vi "UltrasonicRead.vi"(0 "DIO Reference":T1, 1 "TimeoutMS":dbl, 3 "error in (no error)":errorcluster) -> (7 "DistanceM":dbl, 8 "Timeout":bool, 10 "error out":errorcluster)   [LabVIEW 2017]
uses:
  <vilib>/myRIO/Instrument Drivers/Onboard IO/DIO/typedefs/DIO Reference.ctl
  <vilib>/myRIO/Common/Instrument Driver Framework/Utilities/typedefs/myRIO Generic Hardware Reference.ctl
  <vilib>/myRIO/Common/Instrument Driver Framework/Utilities/typedefs/Hardware Version Enum.ctl
  <vilib>/myRIO/Common/Instrument Driver Framework/Utilities/typedefs/myRIO v1.0 Reference.ctl
  <vilib>/myRIO/Common/Instrument Driver Framework/Utilities/typedefs/Generic FPGA Reference.ctl
  <vilib>/myRIO/Common/Instrument Driver Framework/myRIO v1.0/DIO/typedefs/DIO Channels List.ctl
  <vilib>/myRIO/Common/Instrument Driver Framework/myRIO v1.0/DIO/typedefs/DIO Channels Enum.ctl
  <vilib>/Utility/error.llb/Error Cluster From Error Code.vi
  <vilib>/myRIO/Common/Instrument Driver Framework/myRIO v1.0/DIO/vis/myRIO v1.0 Write DIO.vi
  <vilib>/myRIO/Common/Instrument Driver Framework/myRIO v1.0/DIO/vis/myRIO v1.0 Read DIO.vi
  <vilib>/myRIO/Instrument Drivers/Onboard IO/DIO/DIO.lvlib
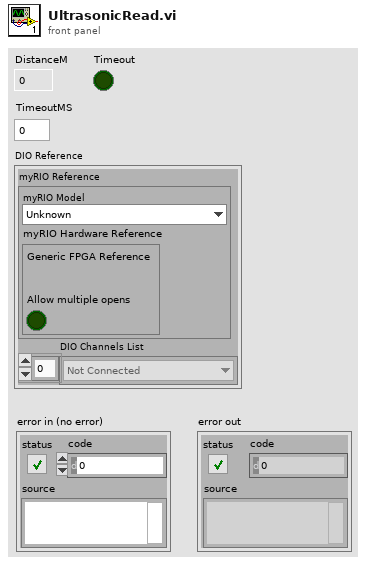
[diagram p1: front panel]
types:
  T1 = typedef "DIO.lvlib/DIO Reference.ctl" = cluster{"myRIO Reference":T2, "DIO Channels List":T6}
  T2 = typedef "myRIO Generic Hardware Reference.ctl" = cluster{"myRIO Model":T3, "myRIO Hardware Reference":T4}
  T3 = typedef "Hardware Version Enum.ctl" = enum16{"Unknown", "myRIO-1900", "myRIO-1950", "roboRIO", "NI ELVIS RIO CM"}
  T4 = typedef "myRIO v1.0 Reference.ctl" = cluster{"Generic FPGA Reference":T5, "Allow multiple opens":bool}
  T5 = typedef "Generic FPGA Reference.ctl" = refnum<k20>
  T6 = typedef "DIO Channels List.ctl" = T7[]
  T7 = typedef "DIO Channels Enum.ctl" = enum16{"Not Connected", "C/DIO0", "C/DIO1", "C/DIO2", "C/DIO3", "C/DIO4", "C/DIO5", "C/DIO6", "C/DIO7", "A/DIO0", "A/DIO1", "A/DIO2", "A/DIO3", "A/DIO4", "A/DIO5", "A/DIO6", "A/DIO7", "A/DIO8", "A/DIO9", "A/DIO10", "A/DIO11", "A/DIO12", "A/DIO13", "A/DIO14", "A/DIO15", "B/DIO0", "B/DIO1", "B/DIO2", "B/DIO3", "B/DIO4", "B/DIO5", "B/DIO6", "B/DIO7", "B/DIO8", "B/DIO9", "B/DIO10", "B/DIO11", "B/DIO12", "B/DIO13", "B/DIO14", "B/DIO15", "LED0", "LED1", "LED2", "LED3", "Button0", "DIO/DIO0", "DIO/DIO1", "DIO/DIO2", "DIO/DIO3", "DIO/DIO4", "DIO/DIO5", "DIO/DIO6", "DIO/DIO7", "DIO/DIO8", "DIO/DIO9", "SPI/CS0", "SPI/CS1", "SPI/CS2", "SPI/CS3", "LED RADIO (Green)", "LED RADIO (Red)", "LED COMM (Green)", "LED COMM (Red)", "LED MODE (Green)", "LED MODE (Red)"}
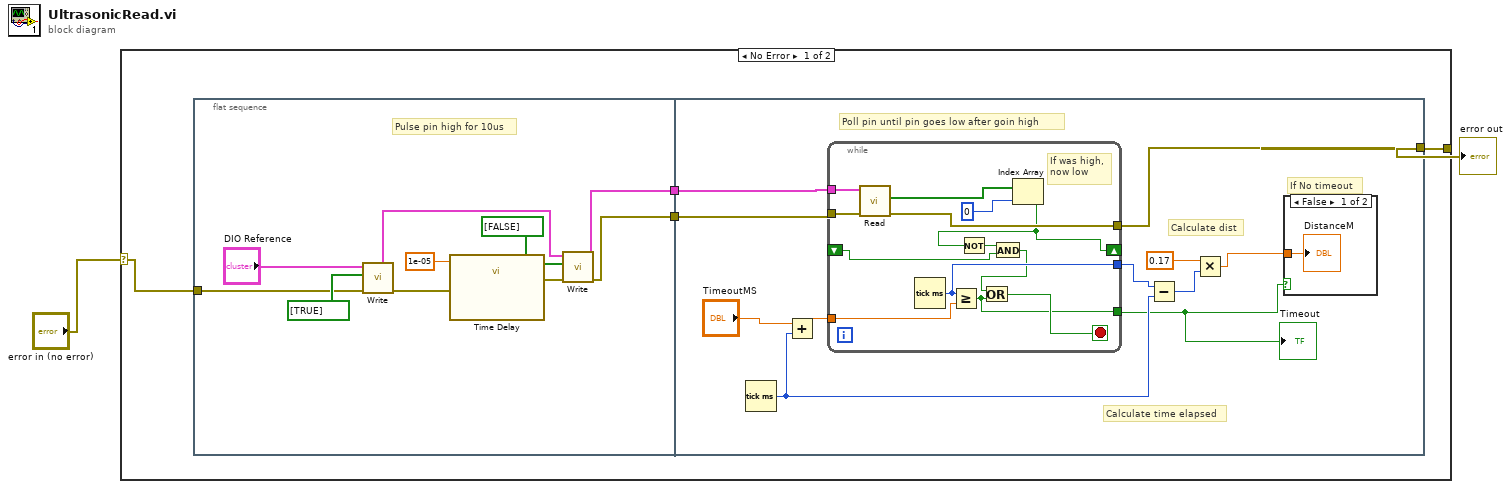
[diagram p0: block diagram]
diagram:
  n1 = case shown="No Error" "error in (no error)" {
    selector: "error in (no error)" -> [w3 w42]
    tunnel: [w4 w42] -> w1
    frame No Error {
      n2 = flat-sequence {
        tunnel: [w9] -> w6
        tunnel: [w8] -> w5
        tunnel: w3 -> [w7]
        tunnel: w6 -> [w25]
        tunnel: w5 -> [w24]
        tunnel: [w23] -> w4
        frame #0 {
          # "Pulse pin high for 10us"
          n3 = call <vilib>:"Write.vi"("error in (no error)"=w7, "Values"=bool[] [TRUE], "DIO Ref In"="DIO Reference") -> ("error out"=w13:errorcluster, "DIO Ref Out"=w10:T1)  [unwired: 6 in]
          n4 = call "Time Delay"("error in (no error)"=w13, "Delay Time (s)"=1e-05) -> ("error out"=w11:errorcluster)  [unwired: 9 in]
          n5 = call <vilib>:"Write.vi"("error in (no error)"=w11, "Values"=bool[] [FALSE], "DIO Ref In"=w10) -> ("error out"=w8:errorcluster, "DIO Ref Out"=w9:T1)  [unwired: 6 in]
        }
        frame #1 {
          # "Calculate time elapsed"
          # "Calculate dist"
          # "Poll pin until pin goes low after goin high"
          # "If No timeout"
          n6 = Tick Count (ms)() -> (millisecond timer value=w21:u32)
          n7 = Add(x="TimeoutMS", y=w21) -> (x+y=w27:dbl)
          n8 = while {
            tunnel: w27 -> [w41]
            tunnel: w25 -> [w38]
            tunnel: w24 -> [w37]
            tunnel: [w39] -> w20
            tunnel: [w36] -> w23
            tunnel: [w33] -> w17
            shift-right: [w32] -> _
            shift-left: _ -> [w30]
            stop <- w40 stop-if-true
            # "If was high,\nnow low"
            n9 = call <vilib>:"Read.vi"("error in (no error)"=w37, "DIO Ref In"=w38) -> ("error out"=w36:errorcluster, "Values"=w35:bool[])  [unwired: 7 in, 1 out]
            n10 = Tick Count (ms)() -> (millisecond timer value=w39:u32)
            n11 = Greater Or Equal?(x=w39, y=w41) -> (x >= y?=w33:bool)
            n12 = Index Array(array=w35, index=0) -> (element=w32:bool)
            n13 = Not(x=w32) -> (.not. x?=w31:bool)
            n14 = And(x=w31, y=w30) -> (x .and. y?=w29:bool)
            n15 = Or(x=w29, y=w33) -> (x .or. y?=w40:bool)
          }
          "Timeout" <- w17
          n16 = Subtract(x=w20, y=w21) -> (x-y=w22:u32)
          n17 = Multiply(x=0.17, y=w22) -> (x*y=w18:dbl)
          n18 = case shown="False" w17 {
            tunnel: w18 -> [w28 _]
            frame False {
              "DistanceM" <- w28
            }
            frame True {
            }
          }
        }
      }
    }
    frame Error {
    }
  }
  "error out" <- w1
